vi "Validate Python Name.vi"(8 "error in (no error)":errorcluster, 11 "Name In":string) -> (0 "error out":errorcluster, 3 "Valid Name":string)   [LabVIEW 2021, in "CIFCoreCommon.lvlib"]
uses:
  CIFCoreCommon.lvlib
  Typedef/Errors.ctl
  <vilib>/CIF Foundation/CIF Utilities/Errors/Append Error Location.vi
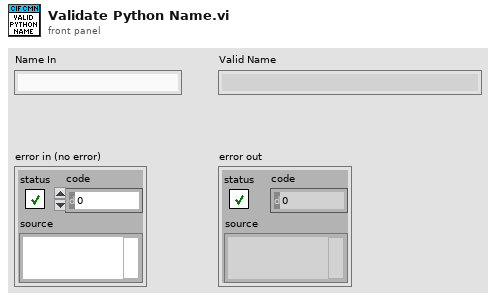
[diagram p1: front panel]
types:
  T1 = typedef "CIFCoreCommon.lvlib/Errors.ctl" = enum16{"Invalid Clock ID", "Long Sleep", "gRPC Server Not Found", "Config Parse", "Timestamp Wrap", "Delayed Execution", "Duplicate Channel", "Missing Channel", "Incorrect Type", "Flatten Error", "Unflatten Data", "Unique Name", "Plugin Not Found", "Plugin Type Not Found", "Plugin Version Not Found", "Manager Not Found", "Numerical Issue", "Time Jump", "Clock ID Match", "Channel Length", "Plugin Connection", "gRPC Server Connection", "PPL Name Match", "Build", "Config Log Parse", "Plugin Load", "UI Subpanel Load", "Python Name", "Invalid Name"}
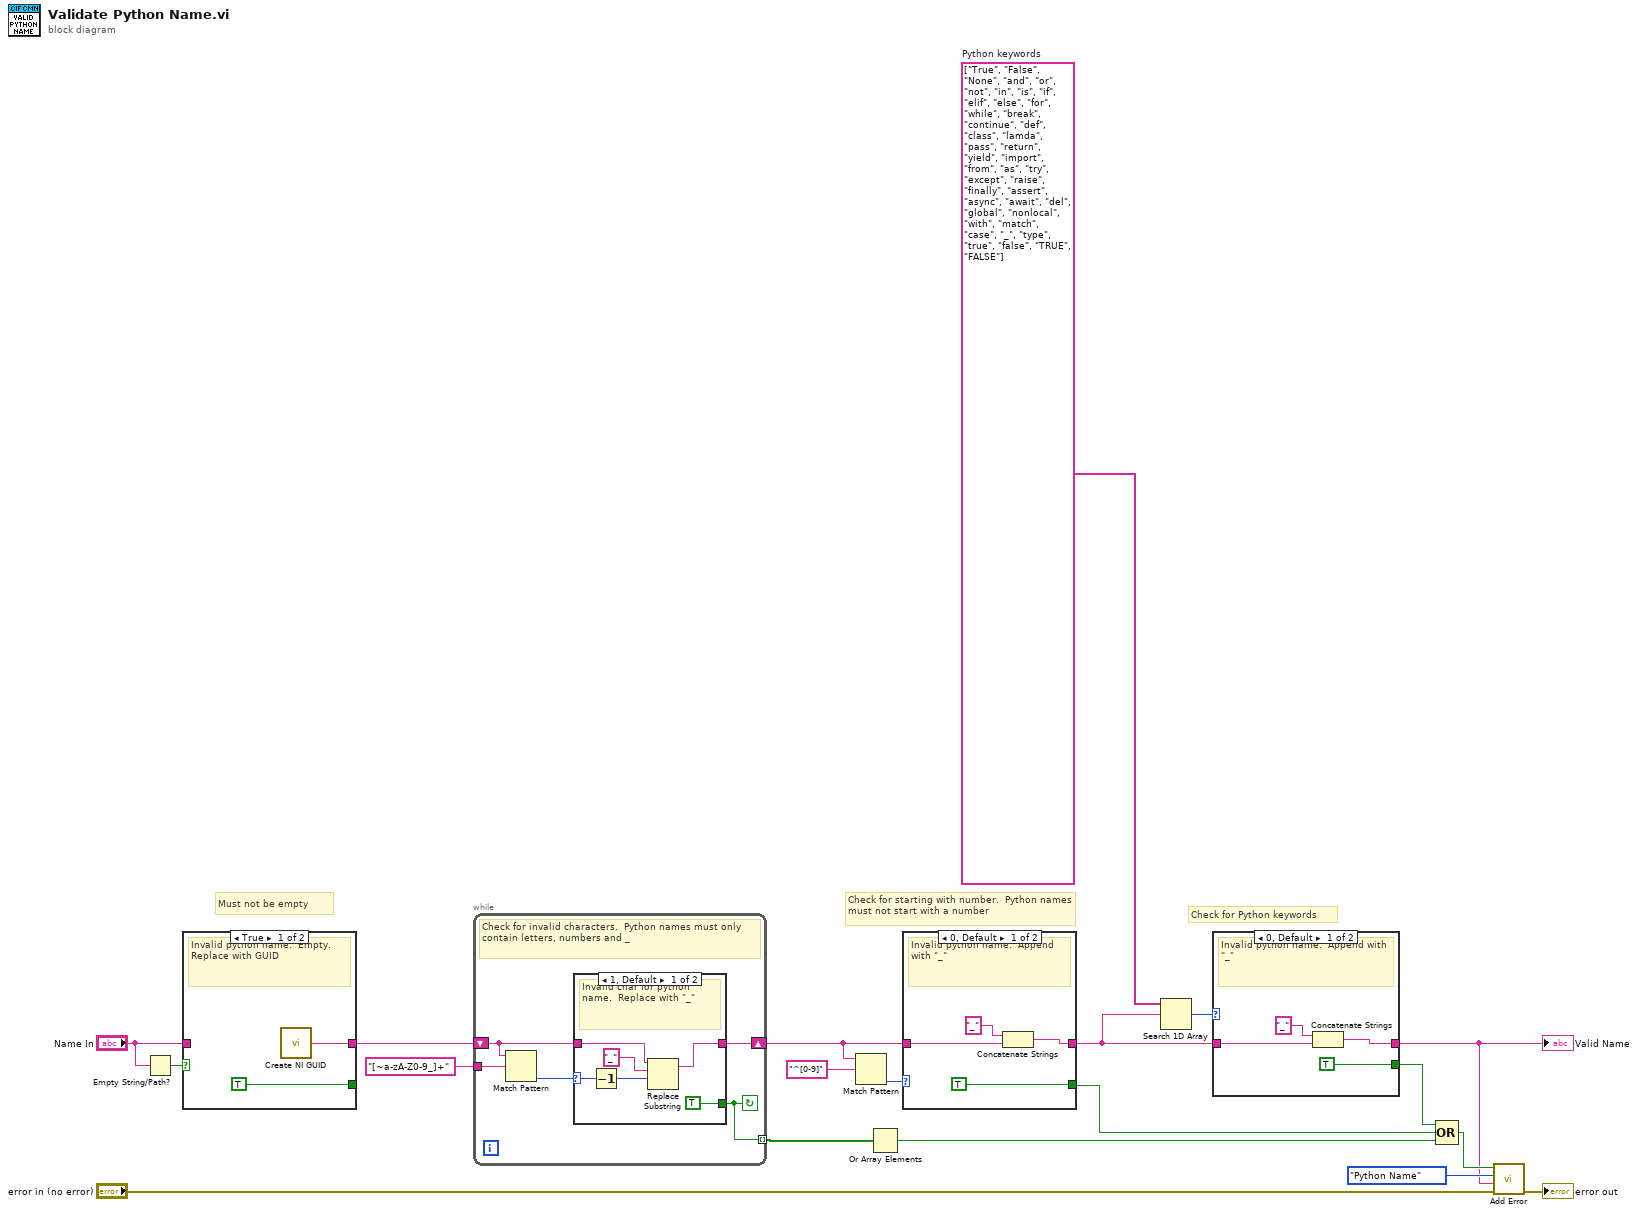
[diagram p0: block diagram]
diagram:
  w16 = string[] ["True", "False", "None", "and", "or", "not", "in", "is", "if", "elif", "else", "for", "while", "break", "continue", "def", "class", "lamda", "pass", "return", "yield", "import", "from", "as", "try", "except", "raise", "finally", "assert", "async", "await", "del", "global", "nonlocal", "with", "match", "case", "_", "type", "true", "false", "TRUE", "FALSE"]  # Python keywords
  # "Must not be empty"
  # "Check for Python keywords"
  # "Check for starting with number.  Python names must not start with a number"
  n1 = Empty String/Path?(string/path="Name In") -> (empty?=w1:bool)
  n2 = case shown="True" w1 {
    tunnel: [w20 w22] -> w3
    tunnel: "Name In" -> [_ w22]
    tunnel: [TRUE _] -> _
    frame True {
      # "Invalid python name.  Empty.  Replace with GUID"
      n3 = call <vilib>:"Create NI GUID.vi"() -> ("NI GUID"=w20:string)
    }
    frame False {
      # "Valid"
    }
  }
  n4 = while {
    tunnel: "[~a-zA-Z0-9_]+" ("regular expression") -> [w27]
    shift-right: [w24] -> w13
    shift-left: w3 -> [w25]
    tunnel: [w23] -> w12 mode=indexing
    stop <- w23 continue-if-true
    # "Check for invalid characters.  Python names must only contain letters, numbers and _"
    n5 = Match Pattern(string=w25, regular expression=w27) -> (offset past match=w26:i32)  [unwired: 1 in, 3 out]
    n6 = case shown="1, Default" w26 {
      selector: w26 -> [w31 _]
      tunnel: w25 -> [w30 w34]
      tunnel: [w29 w34] -> w24
      tunnel: [TRUE _] -> w23
      frame 1, Default {
        # "Invalid char for python name.  Replace with \"_\""
        n7 = Decrement(x=w31) -> (x-1=w33:i32)
        n8 = Replace Substring(3:w33, 4:"_" ("substring (\"\")"), 5:w30) -> (1:w29:string)  [unwired: 1 in, 1 out]
      }
      frame -1, 0 {
      }
    }
  }
  n9 = Match Pattern(string=w13, regular expression="^[0-9]") -> (offset past match=w18:i32)  [unwired: 1 in, 3 out]
  n10 = Or Array Elements(Boolean array=w12) -> (logical OR=w9:bool)
  n11 = case shown="0, Default" w18 {
    tunnel: [w36 w39] -> w14
    tunnel: w13 -> [w38 w39]
    tunnel: [TRUE _] -> w11
    frame 0, Default {
      # "Invalid python name.  Append with \"_\""
      n12 = Concatenate Strings("_" ("string"), w38) -> (w36:string)
    }
    frame -1 {
      # "Valid"
    }
  }
  n13 = Search 1D Array(1D array=w16, element=w14) -> (index of element=w15:i32)  [unwired: 1 in]
  n14 = case shown="0, Default" w15 {
    tunnel: [w41 w44] -> w4
    tunnel: w14 -> [w43 w44]
    tunnel: [TRUE _] -> w10
    frame 0, Default {
      # "Invalid python name.  Append with \"_\""
      n15 = Concatenate Strings("_" ("string"), w43) -> (w41:string)
    }
    frame -1 {
      # "Valid"
    }
  }
  "Valid Name" <- w4
  n16 = Compound Arithmetic op=OR(w10, w11, w9) -> (w5:bool)
  n17 = call "Add Error.vi"("error in (no error)"="error in (no error)", "String to Append"=w4, "Error"=Errors."Python Name", "Insert Error"=w5) -> ("error out"=→"error out":errorcluster)  [unwired: 7 in]
